vi "niRFUtil MT UTIL IQ Impairments Quadrature Skew.vi"(0 "Waveform In":T1={"x0"=0.0, "dx"=1.0, "y"=[]} caption="input complex waveform" {"y" format="%.2f"; "dx" format="%^.2e"; "x0" format="%^.2e"}, 2 "Quadrature Skew, deg":dbl format="%.2f", 11 "error in (no error)":errorcluster) -> (4 "Waveform Out":T1 caption="output complex waveform" {"y" format="%.2f"; "dx" format="%^.2e"; "x0" format="%^.2e"}, 15 "error out":errorcluster)   [LabVIEW 2015, in "niRFUtil.lvlib"]
doc: "Performs the Quadrature Skew operation for IQ Impairment of an Input Data Waveform."
uses:
  niRFUtil.lvlib
  Includes/niRFUtil INC Complex Waveform.ctl
  Includes/niRFUtil INC Complex Array.ctl
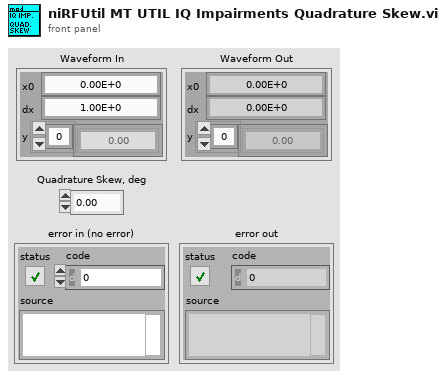
[diagram p1: front panel]
types:
  T1 = typedef "niRFUtil.lvlib/niRFUtil INC Complex Waveform.ctl" = cluster{"x0":dbl, "dx":dbl, "y":T2}
  T2 = typedef "niRFUtil.lvlib/niRFUtil INC Complex Array.ctl" = csg[]
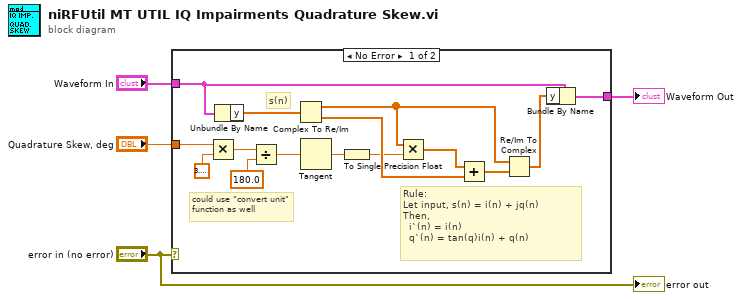
[diagram p0: block diagram]
diagram:
  n1 = case shown="No Error" "error in (no error)" {
    tunnel: "Quadrature Skew, deg" -> [w7 _]
    tunnel: "Waveform In" -> [w18 w20]
    tunnel: [w17 w20] -> w1
    frame No Error {
      # "s(n)"
      # "Rule:\nLet input, s(n) = i(n) + jq(n)\nThen,\n  i`(n) = i(n)\n  q`(n) = tan(q)i(n) + q(n)"
      # "could use \"convert unit\" function as well"
      n2 = Multiply(x=w7, y=3.141592653589793) -> (x*y=w15:dbl)
      n3 = Unbundle By Name(w18) -> ("y"=w19:T2)
      n4 = Divide(x=w15, y=180.0) -> (x/y=w9:dbl)
      n5 = Complex To Re/Im(x + iy=w19) -> (x=w12:sgl[], y=w6:sgl[])
      n6 = Tangent(1:w9) -> (0:w8:dbl)
      n7 = To Single Precision Float(number=w8) -> (single precision float=w5:sgl)
      n8 = Multiply(x=w12, y=w5) -> (x*y=w11:sgl[])
      n9 = Add(x=w11, y=w6) -> (x+y=w10:sgl[])
      n10 = Re/Im To Complex(1:w10, 2:w12) -> (0:w16:csg[])
      n11 = Bundle By Name(cluster=w18, "y"=w16) -> (w17:T1)
    }
    frame Error {
    }
  }
  "Waveform Out" <- w1
  "error out" <- "error in (no error)"
